vi "New One-Shot Subscription.vi"(10 "Ignore Past Updates? (F)":bool, 11 "OneShotSubscription In":refnum<class "OneShotSubscription.lvclass">) -> (3 "OneShotSubscription Out":refnum<class "OneShotSubscription.lvclass">)   [LabVIEW 2020, in "SubscriptionPolicy.lvlib" / "OneShotSubscription.lvclass"]
uses:
  <vilib>/gpm_packages/@cs/mva-core/Source/SubscriptionPolicy/OneShotSubscription/OneShotSubscription.lvclass
  <vilib>/gpm_packages/@cs/mva-core/Source/SubscriptionPolicy/OneShotSubscription/OneShotSubscription.lvclass/OneShotSubscription.ctl
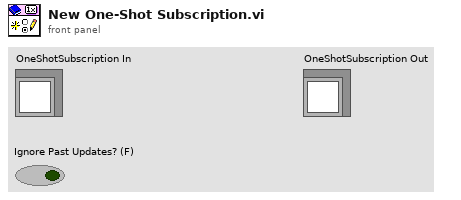
[diagram p1: front panel]
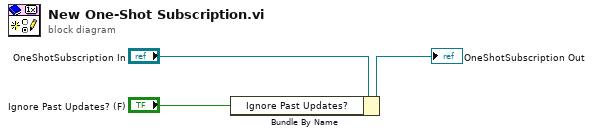
[diagram p0: block diagram]
diagram:
  n1 = Bundle By Name(cluster="OneShotSubscription In", "Ignore Past Updates?"="Ignore Past Updates? (F)") -> (→"OneShotSubscription Out":refnum<class "OneShotSubscription.lvclass">)
